vi "Configure Acquisition Type.vi"(8 "error in (no error)":errorcluster, 9 "Number of Averaged Waveforms (4: 4)":i32(ring)=4 items=["4"=4, "16"=16, "64"=64, "128"=128], 10 "Acquisition Type (0: Sample)":i32(ring) items=["Sample", "Average", "Peak Detect"], 11 "VISA resource name":refnum<visa-resource-name>) -> (0 "error out":errorcluster, 3 "VISA resource name out":refnum<visa-resource-name>)   [LabVIEW 2015, in "Tektronix TDS 200 1000 2000 Series.lvlib"]
doc: "Configures the amount and type of data the oscilloscope acquires from waveforms."
uses:
  <instrlib>/Tektronix TDS 200 1000 2000 Series/Tektronix TDS 200 1000 2000 Series.lvlib
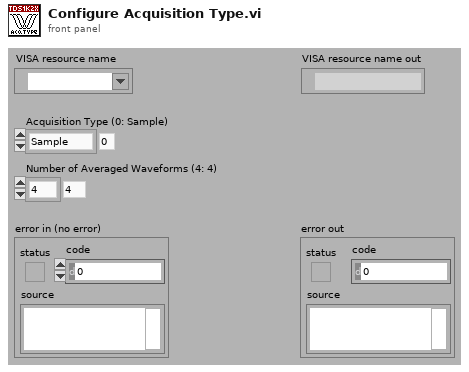
[diagram p1: front panel]
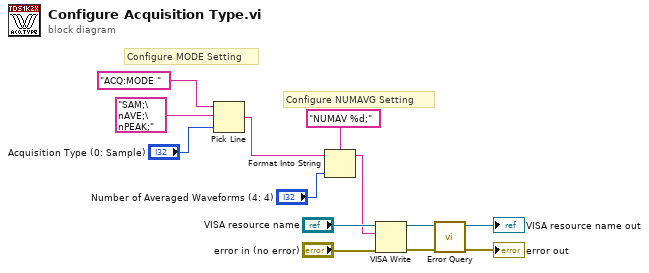
[diagram p0: block diagram]
diagram:
  # "Configure NUMAVG Setting"
  # "Configure MODE Setting"
  n1 = Pick Line(string ("")="ACQ:MODE ", multi-line string="SAM;\nAVE;\nPEAK;", line index="Acquisition Type (0: Sample)") -> (output string=w8:string)
  n2 = Format Into String(format string="NUMAV %d;", initial string=w8, "Number of Averaged Waveforms (4: 4)") -> (resulting string=w1:string)  [unwired: 1 in, 1 out]
  n3 = VISA Write(VISA resource name="VISA resource name", write buffer=w1, error in (no error)="error in (no error)") -> (VISA resource name out=w7:refnum<visa-resource-name>, error out=w6:errorcluster)  [unwired: 1 out]
  n4 = call <instrlib>:"Error Query.vi"("error in (no error)"=w6, "VISA resource name"=w7) -> ("error out"=→"error out":errorcluster, "VISA resource name out"=→"VISA resource name out":refnum<visa-resource-name>)  [unwired: 8 out]
